vi "GetAuditor.vi"() -> (2 "Array":string[](array[string]))   [LabVIEW 2012]
uses:
  <vilib>/addons/database/Auxilliary.llb/DB Tools Cursor Type.ctl
  <vilib>/addons/database/Connection.llb/DB Tools Open Connec (Path).vi
  <vilib>/addons/database/Connection.llb/Conn Execute.vi
  <vilib>/addons/database/Recordset.llb/Rec Fetch String Data (R).vi
  <vilib>/addons/database/Recordset.llb/Rec Destroy - Connection.vi
  <vilib>/addons/database/Recordset.llb/Rec Get Recordset Properties (R).vi
  <vilib>/addons/database/NI_Database_API.lvlib
panel:
  out "Teléfono":string
  out "Apellido":string
  out "Nombre":string
  in  "ID":u16(ring) items=["-", "1", "2", "3"]
  in  "stop":bool
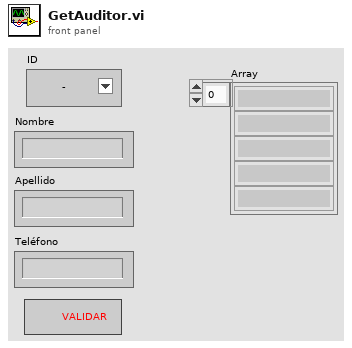
[diagram p1: front panel]
types:
  T1 = typedef "NI_Database_API.lvlib/Conn ObjectReference.ctl" = refnum<k1>
  T2 = typedef "NI_Database_API.lvlib/DB Tools Cursor Type.ctl" = enum16{"forward-only", "keyset", "dynamic", "static"}
  T3 = typedef "NI_Database_API.lvlib/Rec ObjectReference.ctl" = refnum<k1>
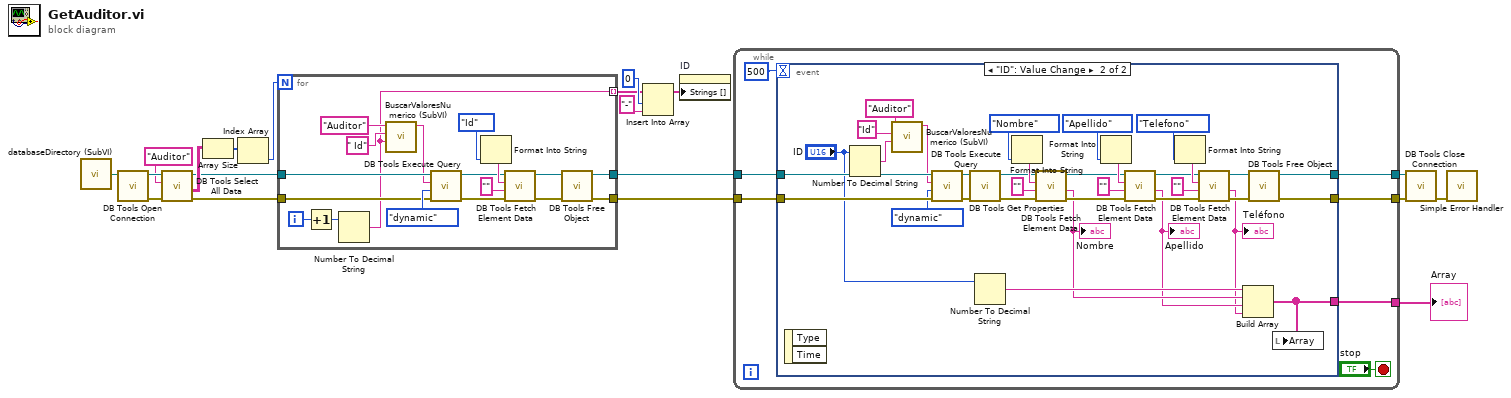
[diagram p0: block diagram]
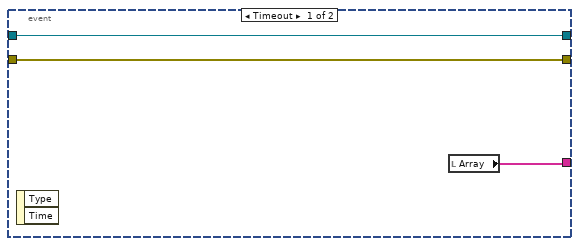
[diagram p2: hidden frame]
diagram:
  n1 = call "databaseDirectory (SubVI).vi"() -> ("Application Directory"=w7:path)  [unwired: 1 in]
  n2 = call-poly <vilib>:"DB Tools Open Connection.vi"("connection information"=w7) -> ("error out"=w12:errorcluster, "connection reference"=w11:T1)  [unwired: 7 in]
  n3 = call <vilib>:"DB Tools Select All Data.vi"("error in (no error)"=w12, "table"="Auditor", "connection reference"=w11) -> ("error out"=w6:errorcluster, "data"=w14:string[][], "connection reference out"=w10:T1)  [unwired: 3 in]
  n4 = Array Size(array=w14) -> (size(s)=w13:i32[])
  n5 = Index Array(array=w13) -> (element=w8:i32)  [unwired: 1 in]
  n6 = for {
    N: w8 -> [_]
    tunnel: w10 -> [w33]
    tunnel: w6 -> [w34]
    tunnel: [w32] -> w4
    tunnel: [w31] -> w3
    tunnel: [w23] -> w5 mode=indexing
    i -> [w22]
    n7 = Increment(x=w22) -> (x+1=w21:i32)
    n8 = Number To Decimal String(number=w21) -> (decimal integer string=w23:string)  [unwired: 1 in]
    n9 = call "BuscarValoresNumerico (SubVI).vi"("="=w23, "Columna"=" Id" ("Substring"), "Tabla"="Auditor" ("table")) -> ("String"=w30:string)  [unwired: 8 in]
    n10 = call-poly <vilib>:"DB Tools Execute Query.vi"("error in (no error)"=w34, "cursor type"=DB_Tools_Cursor_Type."dynamic", "SQL query"=w30, "connection reference"=w33) -> ("error out"=w26:errorcluster, "recordset reference"=w27:T3)  [unwired: 4 in]
    n11 = Format Into String(enum16{"Id", "Nombre", "Apellido", "Telefono"}."Id") -> (resulting string=w37:string)  [unwired: 3 in, 1 out]
    n12 = call-poly <vilib>:"DB Tools Fetch Element Data.vi"("error in (no error)"=w26, "type"="", "column index"=w37, "recordset reference"=w27) -> ("error out"=w24:errorcluster, "recordset reference out"=w25:T3)  [unwired: 3 in, 1 out]
    n13 = call-poly <vilib>:"DB Tools Free Object.vi"("error in (no error)"=w24, "recordset reference"=w25) -> ("error out"=w31:errorcluster, "connection reference"=w32:T1)  [unwired: 8 in]
  }
  n14 = Insert Into Array(array=w5, index=0, new element="-" ("new element/subarray")) -> (w2:string[])
  n15 = property on="ID" class="Ring (strict)"("Strings []"=w2) -> ()  [unwired: 2 in, 2 out]
  n16 = while {
    tunnel: w4 -> [w44]
    tunnel: w3 -> [w43]
    tunnel: [w40] -> w18
    tunnel: [w39] -> w17
    tunnel: [w38] -> w1
    stop <- "stop" stop-if-true
    n17 = event shown="[1] \"ID\": Value Change" {
      selector: _ -> [_ _]
      dyn-events: _ -> [_ _]
      timeout: 500 -> [_ _]
      tunnel: w44 -> [w47 w80]
      tunnel: w43 -> [w46 w81]
      tunnel: [w47 w79] -> w40
      tunnel: [w46 w78] -> w39
      tunnel: [w45 w48] -> w38
      event Timeout {
        n18 = event-data() -> ()  [unwired: 1 in, 2 out]
        n19 = local read "Array"() -> (w45:string[])
      }
      event "ID": Value Change {
        n20 = event-data() -> ()  [unwired: 1 in, 2 out]
        n21 = Number To Decimal String(number="ID") -> (decimal integer string=w63:string)  [unwired: 1 in]
        n22 = call "BuscarValoresNumerico (SubVI).vi"("="=w63, "Columna"="Id" ("Substring"), "Tabla"="Auditor" ("table")) -> ("String"=w68:string)  [unwired: 8 in]
        n23 = call-poly <vilib>:"DB Tools Execute Query.vi"("error in (no error)"=w81, "cursor type"=DB_Tools_Cursor_Type."dynamic", "SQL query"=w68, "connection reference"=w80) -> ("error out"=w74:errorcluster, "recordset reference"=w75:T3)  [unwired: 4 in]
        n24 = call-poly <vilib>:"DB Tools Get Properties.vi"("error in (no error)"=w74, "recordset reference"=w75) -> ("error out"=w64:errorcluster, "recordset reference out"=w65:T3)  [unwired: 3 in, 1 out]
        n25 = Number To Decimal String(number="ID") -> (decimal integer string=w52:string)  [unwired: 1 in]
        n26 = Format Into String(enum16{"Id", "Nombre", "Apellido", "Telefono"}."Nombre") -> (resulting string=w77:string)  [unwired: 3 in, 1 out]
        n27 = call-poly <vilib>:"DB Tools Fetch Element Data.vi"("error in (no error)"=w64, "type"="", "column index"=w77, "recordset reference"=w65) -> ("error out"=w69:errorcluster, "data"=w51:string, "recordset reference out"=w70:T3)  [unwired: 3 in]
        "Nombre" <- w51
        n28 = Format Into String(enum16{"Id", "Nombre", "Apellido", "Telefono"}."Apellido") -> (resulting string=w71:string)  [unwired: 3 in, 1 out]
        n29 = call-poly <vilib>:"DB Tools Fetch Element Data.vi"("error in (no error)"=w69, "type"="", "column index"=w71, "recordset reference"=w70) -> ("error out"=w54:errorcluster, "data"=w50:string, "recordset reference out"=w57:T3)  [unwired: 3 in]
        "Apellido" <- w50
        n30 = Format Into String(enum16{"Id", "Nombre", "Apellido", "Telefono"}."Telefono") -> (resulting string=w59:string)  [unwired: 3 in, 1 out]
        n31 = call-poly <vilib>:"DB Tools Fetch Element Data.vi"("error in (no error)"=w54, "type"="", "column index"=w59, "recordset reference"=w57) -> ("error out"=w55:errorcluster, "data"=w49:string, "recordset reference out"=w56:T3)  [unwired: 3 in]
        "Teléfono" <- w49
        n32 = Build Array(w52, w51, w50, w49) -> (w48:string[])
        n33 = call-poly <vilib>:"DB Tools Free Object.vi"("error in (no error)"=w55, "recordset reference"=w56) -> ("error out"=w78:errorcluster, "connection reference"=w79:T1)  [unwired: 8 in]
        n34 = local write "Array"(w48) -> ()
      }
    }
  }
  "Array" <- w1
  n35 = call <vilib>:"DB Tools Close Connection.vi"("error in (no error)"=w17, "connection reference"=w18) -> ("error out"=w19:errorcluster)  [unwired: 5 in]
  n36 = call <vilib>:"Simple Error Handler.vi"("error in (no error)"=w19) -> ()  [unwired: 4 in, 5 out]
